vi "Edit single ROI overlay.vi"(5 "Selected ?":bool, 6 "Abs. index of selected Z-plane (unity-based)":i32, 7 "Number of Z-planes":i32, 8 "ROI Properties":T1 {"Apparent Frame Size" format="%#_6f"; "Original FOV (um)" format="%#_6f"; "Pixels per miniscan" format="%#_6f"; "Dwell Time per pixel" format="%#_6f"; "Resolution" format="%#_6f"; "ROI group ID" format="%#_6f"; "Laser Power (%)" format="%#_6f"; "Zoom" format="%#_6f"; "Frame Size" format="%#_6f"; "Number of lines" format="%#_6f"; "Composite ID" format="%#_6f"; "Angle (deg)" format="%#_6f"; "ROI Time (ns)" format="%#_6f"; "ROI ID" format="%#_6f"; "Pixels in ROI" format="%#_6f"; "ROI index" format="%#_6f"; "Z stop" format="%#_6f"; "Y stop" format="%#_6f"; "X stop" format="%#_6f"; "Z start" format="%#_6f"; "X start" format="%#_6f"; "Y start" format="%#_6f"}, 9 "Z code":u8, 10 "Image2":T2, 11 "Image1":T2) -> (0 "Error out":errorcluster, 2 "Image2 Out":T2, 3 "Image1 Out":T2)   [LabVIEW 2020]
uses:
  <vilib>/vision/Image Controls.llb/IMAQ Image.ctl
  Typedefs/ROI parameters data type.ctl
panel:
  in  "Volume Colour":u32(colorbox)=27903
  in  "Rectangular text Colour":u32(colorbox)=6618880
  in  "Rectangular line Colour":u32(colorbox)=56063
  in  "POI text Colour":u32(colorbox)=6618880
  in  "Miniscan text colour":u32(colorbox)=6618880
  in  "POI line Colour":u32(colorbox)=16711680
  in  "Miniscan line colour":u32(colorbox)=16682774
  in  "Text Colour":u32(colorbox)=13882323
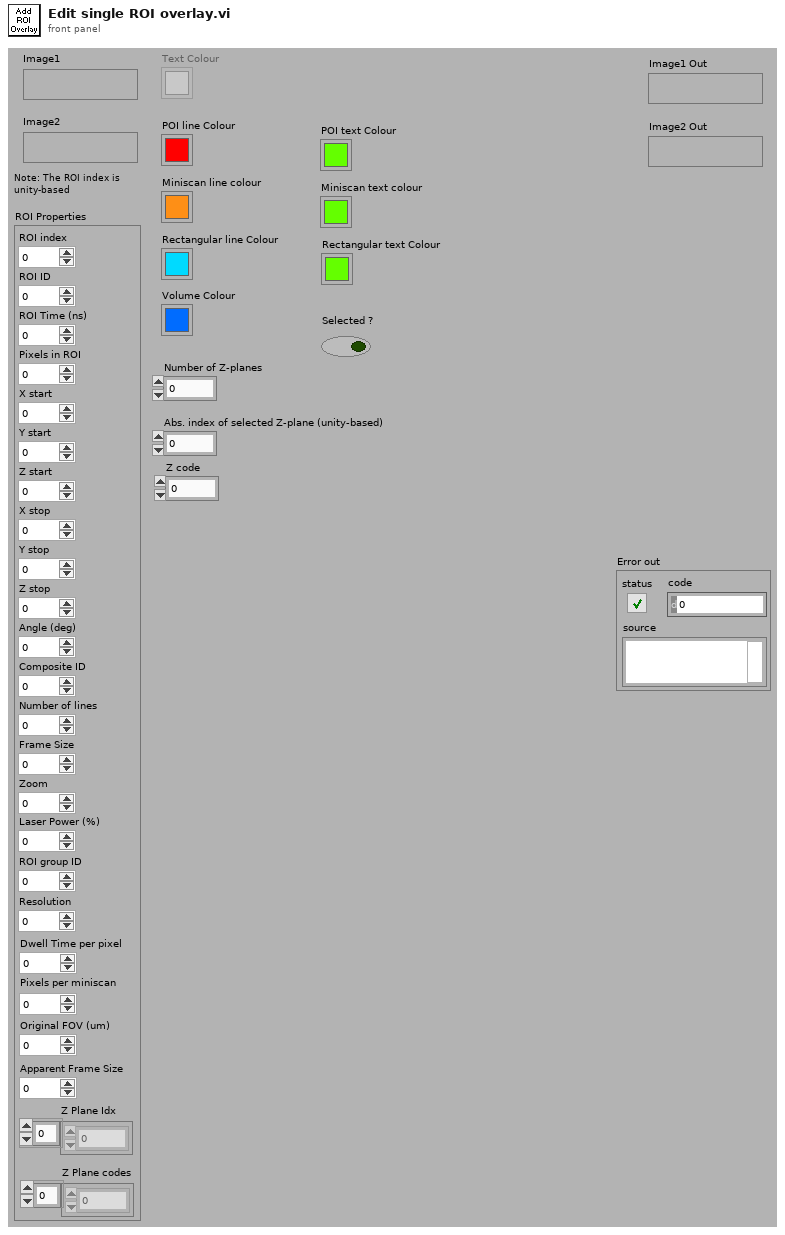
[diagram p1: front panel]
types:
  T1 = typedef "ROI parameters data type.ctl" = cluster{"ROI index":dbl, "ROI ID":dbl, "ROI Time (ns)":dbl, "Pixels in ROI":dbl, "X start":dbl, "Y start":dbl, "Z start":dbl, "X stop":dbl, "Y stop":dbl, "Z stop":dbl, "Angle (deg)":dbl, "Composite ID":dbl, "Number of lines":dbl, "Frame Size":dbl, "Zoom":dbl, "Laser Power (%)":dbl, "ROI group ID":dbl, "Resolution":dbl, "Dwell Time per pixel":dbl, "Pixels per miniscan":dbl, "Original FOV (um)":dbl, "Apparent Frame Size":dbl, "Z Plane Idx":i32[], "Z Plane codes":i32[]}
  T2 = typedef "IMAQ Image.ctl" = refnum<image>
  T3 = cluster{"Left":i32, "Top":i32, "Right":i32, "Bottom":i32}
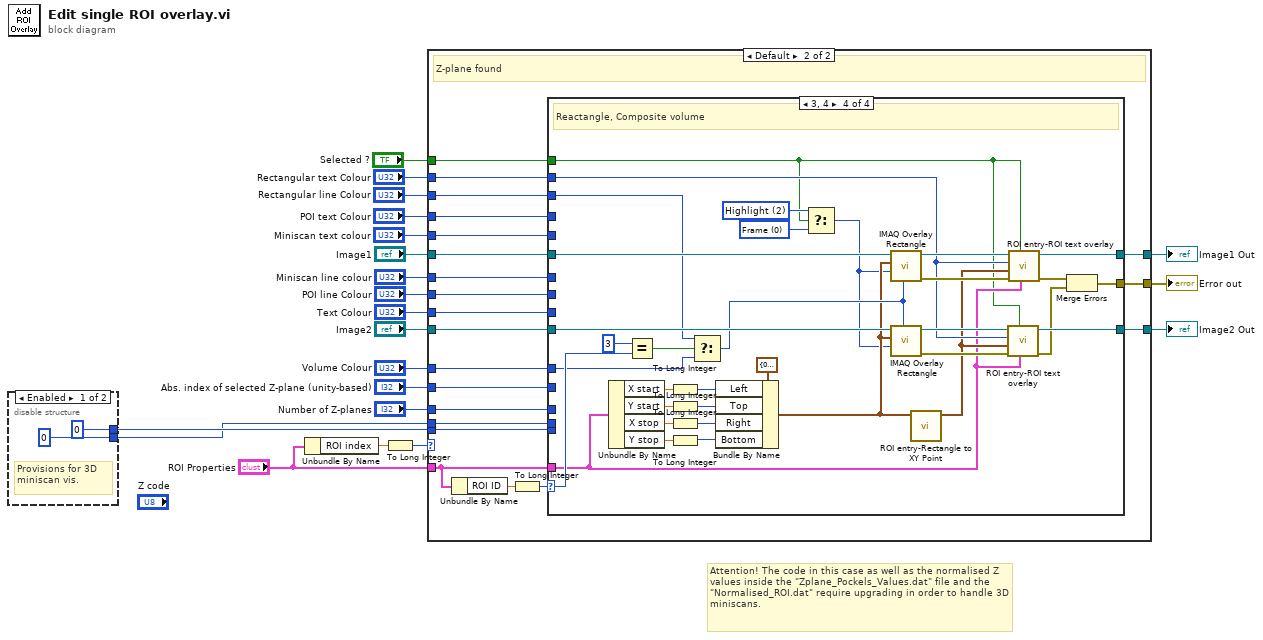
[diagram p0: block diagram]
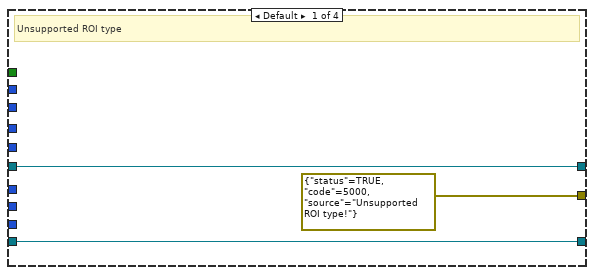
[diagram p4: hidden frame]
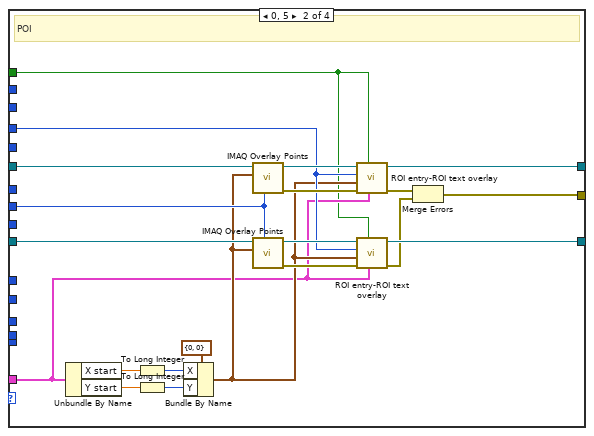
[diagram p5: hidden frame]
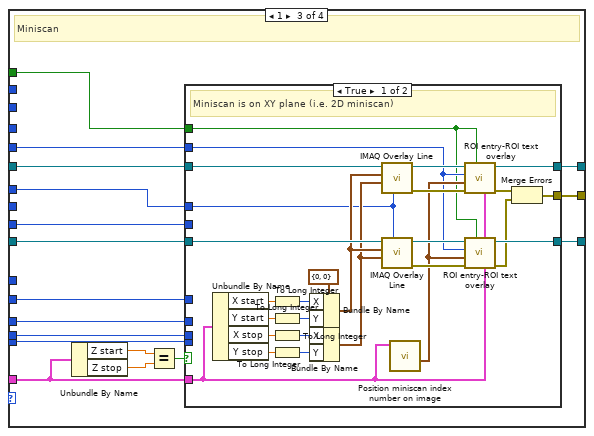
[diagram p6: hidden frame]
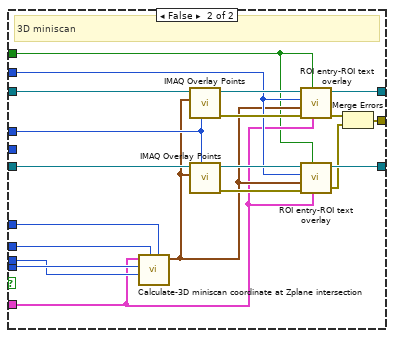
[diagram p7: hidden frame]
diagram:
  # "Attention! The code in this case as well as the normalised Z values inside the \"Zplane_Pockels_Values.dat\" file and the \"Normalised_ROI.dat\" require upgrading in order to handle 3D miniscans."
  n1 = disable-structure "Diagram Disable Structure" shown="Enabled" {
    disable-tunnel: [0 ("Number of intersected Zplanes") _] -> w12
    disable-tunnel: [0 ("Number of intersected Zplanes") _] -> w11
    frame Enabled {
      # "Provisions for 3D miniscan vis."
    }
    frame Disabled {
    }
  }
  n2 = Unbundle By Name("ROI Properties") -> ("ROI index"=w17:dbl)
  n3 = To Long Integer(number=w17) -> (32bit integer=w2:i32)
  n4 = case shown="Default" w2 {
    tunnel: "Image1" -> [w25 w46]
    tunnel: "Image2" -> [w24 w45]
    tunnel: [w25 w44] -> w20
    tunnel: [w24 w43] -> w19
    tunnel: "ROI Properties" -> [_ w41]
    tunnel: "Text Colour" -> [_ w40]
    tunnel: "Number of Z-planes" -> [_ w38]
    tunnel: "Abs. index of selected Z-plane (unity-based)" -> [_ w39]
    tunnel: w12 -> [_ w37]
    tunnel: w11 -> [_ w36]
    tunnel: "POI line Colour" -> [_ w35]
    tunnel: "Miniscan line colour" -> [_ w34]
    tunnel: "Miniscan text colour" -> [_ w33]
    tunnel: "POI text Colour" -> [_ w32]
    tunnel: [_ w31] -> w6
    tunnel: "Rectangular text Colour" -> [_ w30]
    tunnel: "Rectangular line Colour" -> [_ w29]
    tunnel: "Volume Colour" -> [_ w28]
    tunnel: "Selected ?" -> [_ w26]
    frame -1 {
      # "Z-plane not found"
    }
    frame Default {
      # "Z-plane found"
      n5 = Unbundle By Name(w41) -> ("ROI ID"=w42:dbl)
      n6 = To Long Integer(number=w42) -> (32bit integer=w27:i32)
      n7 = case shown="3, 4" w27 {
        selector: w27 -> [_ _ _ w156]
        tunnel: w46 -> [w49 w66 w87 w168]
        tunnel: w45 -> [w48 w65 w86 w167]
        tunnel: [w49 w64 w85 w149] -> w44
        tunnel: [w48 w63 w84 w145] -> w43
        tunnel: w41 -> [_ w51 w72 w139]
        tunnel: w40 -> [_ _ w80 _]
        tunnel: w39 -> [_ _ w79 _]
        tunnel: w38 -> [_ _ w78 _]
        tunnel: w37 -> [_ _ w77 _]
        tunnel: w36 -> [_ _ w76 _]
        tunnel: w35 -> [_ w56 _ _]
        tunnel: w34 -> [_ _ w75 _]
        tunnel: w33 -> [_ _ w74 _]
        tunnel: w32 -> [_ w57 _ _]
        tunnel: [errorcluster {"status"=TRUE, "code"=5000, "source"="Unsupported ROI type!"} ("error IO") w53 w73 w166] -> w31
        tunnel: w30 -> [_ _ _ w144]
        tunnel: w29 -> [_ _ _ w152]
        tunnel: w28 -> [_ _ _ w153]
        tunnel: w26 -> [_ w50 w71 w137]
        frame Default {
          # "Unsupported ROI type"
        }
        frame 0, 5 {
          # "POI"
          n8 = Unbundle By Name(w51) -> ("X start"=w61:dbl, "Y start"=w60:dbl)
          n9 = To Long Integer(number=w61) -> (32bit integer=w59:i32)
          n10 = To Long Integer(number=w60) -> (32bit integer=w58:i32)
          n11 = Bundle By Name(cluster=cluster{"X":i32, "Y":i32} {"X"=0, "Y"=0} ("Point"), "X"=w59, "Y"=w58) -> (w52:cluster{"X":i32, "Y":i32})
          n12 = call "IMAQ Overlay Points"("Color"=w56, "Point"=w52, "Image"=w66) -> ("error out"=w67:errorcluster, "Image Out"=w68:T2)  [unwired: 7 in]
          n13 = call "IMAQ Overlay Points"("Color"=w56, "Point"=w52, "Image"=w65) -> ("error out"=w70:errorcluster, "Image Out"=w69:T2)  [unwired: 7 in]
          n14 = call "ROI entry-ROI text overlay.vi"("ROI properties"=w51, "Selected ?"=w50, "Error in (no error)"=w67, "Point"=w52, "Rect. text colour"=w57, "Refnum in"=w68) -> ("error out"=w55:errorcluster, "Refnum out"=w64:T2)  [unwired: 4 in]
          n15 = call "ROI entry-ROI text overlay.vi"("ROI properties"=w51, "Selected ?"=w50, "Error in (no error)"=w70, "Point"=w52, "Rect. text colour"=w57, "Refnum in"=w69) -> ("error out"=w54:errorcluster, "Refnum out"=w63:T2)  [unwired: 4 in]
          n16 = Merge Errors(w55, w54) -> (w53:errorcluster)
        }
        frame 1 {
          # "Miniscan"
          n17 = Unbundle By Name(w72) -> ("Z start"=w83:dbl, "Z stop"=w82:dbl)
          n18 = Equal?(x=w83, y=w82) -> (x = y?=w81:bool)
          n19 = case shown="True" w81 {
            tunnel: w87 -> [w110 w130]
            tunnel: w86 -> [w109 w129]
            tunnel: [w108 w128] -> w85
            tunnel: [w107 w127] -> w84
            tunnel: w72 -> [w89 w116]
            tunnel: w75 -> [w94 w121]
            tunnel: w80 -> [_ _]
            tunnel: w79 -> [_ w126]
            tunnel: w78 -> [_ w125]
            tunnel: w77 -> [_ w124]
            tunnel: w76 -> [_ w123]
            tunnel: w74 -> [w93 w122]
            tunnel: [w91 w118] -> w73
            tunnel: w71 -> [w88 w115]
            frame True {
              w105 = cluster{"X":i32, "Y":i32} {"X"=0, "Y"=0} ("Point")
              # "Miniscan is on XY plane (i.e. 2D miniscan)"
              n20 = Unbundle By Name(w89) -> ("X start"=w95:dbl, "Y start"=w96:dbl, "X stop"=w97:dbl, "Y stop"=w98:dbl)
              n21 = To Long Integer(number=w95) -> (32bit integer=w103:i32)
              n22 = To Long Integer(number=w96) -> (32bit integer=w101:i32)
              n23 = To Long Integer(number=w97) -> (32bit integer=w100:i32)
              n24 = To Long Integer(number=w98) -> (32bit integer=w102:i32)
              n25 = Bundle By Name(cluster=w105, "X"=w103, "Y"=w101) -> (w106:cluster{"X":i32, "Y":i32})
              n26 = Bundle By Name(cluster=w105, "X"=w100, "Y"=w102) -> (w104:cluster{"X":i32, "Y":i32})
              n27 = call "IMAQ Overlay Line"("Color"=w94, "End Point"=w104, "Start Point"=w106, "Image"=w110) -> ("error out"=w111:errorcluster, "Image Out"=w112:T2)  [unwired: 6 in]
              n28 = call "IMAQ Overlay Line"("Color"=w94, "End Point"=w104, "Start Point"=w106, "Image"=w109) -> ("error out"=w114:errorcluster, "Image Out"=w113:T2)  [unwired: 6 in]
              n29 = call "Position miniscan index number on image.vi"("X-Y-Z coordinates"=w89) -> ("X-Y coordinates at miniscan middle point"=w99:cluster{"X":i32, "Y":i32})  [unwired: 10 in]
              n30 = call "ROI entry-ROI text overlay.vi"("ROI properties"=w89, "Selected ?"=w88, "Error in (no error)"=w111, "Point"=w99, "Rect. text colour"=w93, "Refnum in"=w112) -> ("error out"=w92:errorcluster, "Refnum out"=w108:T2)  [unwired: 4 in]
              n31 = call "ROI entry-ROI text overlay.vi"("ROI properties"=w89, "Selected ?"=w88, "Error in (no error)"=w114, "Point"=w99, "Rect. text colour"=w93, "Refnum in"=w113) -> ("error out"=w90:errorcluster, "Refnum out"=w107:T2)  [unwired: 4 in]
              n32 = Merge Errors(w92, w90) -> (w91:errorcluster)
            }
            frame False {
              # "3D miniscan"
              n33 = call "Calculate-3D miniscan coordinate at Zplane intersection.vi"("Abs. index of selected Z-plane (unity-based)"=w126, "Number of Z-planes"=w125, "Relative index of selected Z-plane (unity-based)"=w123, "Number of intersected Zplanes"=w124, "input cluster"=w116) -> ("£D miniscan Z-plane intersection coordinates"=w117:cluster{"X":i32, "Y":i32})  [unwired: 6 in]
              n34 = call "IMAQ Overlay Points"("Color"=w121, "Point"=w117, "Image"=w130) -> ("error out"=w131:errorcluster, "Image Out"=w132:T2)  [unwired: 7 in]
              n35 = call "IMAQ Overlay Points"("Color"=w121, "Point"=w117, "Image"=w129) -> ("error out"=w134:errorcluster, "Image Out"=w133:T2)  [unwired: 7 in]
              n36 = call "ROI entry-ROI text overlay.vi"("ROI properties"=w116, "Selected ?"=w115, "Error in (no error)"=w131, "Point"=w117, "Rect. text colour"=w122, "Refnum in"=w132) -> ("error out"=w120:errorcluster, "Refnum out"=w128:T2)  [unwired: 4 in]
              n37 = call "ROI entry-ROI text overlay.vi"("ROI properties"=w116, "Selected ?"=w115, "Error in (no error)"=w134, "Point"=w117, "Rect. text colour"=w122, "Refnum in"=w133) -> ("error out"=w119:errorcluster, "Refnum out"=w127:T2)  [unwired: 4 in]
              n38 = Merge Errors(w120, w119) -> (w118:errorcluster)
            }
          }
        }
        frame 3, 4 {
          w136 = u32 0 items=["Frame", "Fill", "Highlight"] ("Drawing Mode (Frame)")
          w138 = u32 2 items=["Frame", "Fill", "Highlight"] ("Drawing Mode (Frame)")
          # "Reactangle, Composite volume"
          n39 = Unbundle By Name(w139) -> ("X start"=w159:dbl, "Y start"=w163:dbl, "X stop"=w164:dbl, "Y stop"=w165:dbl)
          n40 = Equal?(x=3, y=w156) -> (x = y?=w154:bool)
          n41 = To Long Integer(number=w159) -> (32bit integer=w158:i32)
          n42 = To Long Integer(number=w163) -> (32bit integer=w157:i32)
          n43 = To Long Integer(number=w164) -> (32bit integer=w161:i32)
          n44 = To Long Integer(number=w165) -> (32bit integer=w160:i32)
          n45 = Select(t=w152, s=w154, f=w153) -> (s? t:f=w151:u32)
          n46 = Bundle By Name(cluster=T3 {"Left"=0, "Top"=0, "Right"=0, "Bottom"=0} ("Rectangle"), "Left"=w158, "Top"=w157, "Right"=w161, "Bottom"=w160) -> (w141:T3)
          n47 = Select(t=w138, s=w137, f=w136) -> (s? t:f=w135:u32)
          n48 = call "IMAQ Overlay Rectangle"("Color"=w151, "Drawing Mode (Frame)"=w135, "Rectangle"=w141, "Image"=w168) -> ("error out"=w147:errorcluster, "Image Out"=w150:T2)  [unwired: 6 in]
          n49 = call "IMAQ Overlay Rectangle"("Color"=w151, "Drawing Mode (Frame)"=w135, "Rectangle"=w141, "Image"=w167) -> ("error out"=w142:errorcluster, "Image Out"=w146:T2)  [unwired: 6 in]
          n50 = call "ROI entry-Rectangle to XY Point.vi"("Rectangle"=w141) -> ("XY"=w140:cluster{"X":i32, "Y":i32})  [unwired: 10 in]
          n51 = call "ROI entry-ROI text overlay.vi"("ROI properties"=w139, "Selected ?"=w137, "Error in (no error)"=w142, "Point"=w140, "Rect. text colour"=w144, "Refnum in"=w146) -> ("error out"=w143:errorcluster, "Refnum out"=w145:T2)  [unwired: 4 in]
          n52 = call "ROI entry-ROI text overlay.vi"("ROI properties"=w139, "Selected ?"=w137, "Error in (no error)"=w147, "Point"=w140, "Rect. text colour"=w144, "Refnum in"=w150) -> ("error out"=w148:errorcluster, "Refnum out"=w149:T2)  [unwired: 4 in]
          n53 = Merge Errors(w148, w143) -> (w166:errorcluster)
        }
      }
    }
  }
  "Image1 Out" <- w20
  "Image2 Out" <- w19
  "Error out" <- w6
